vi "flash_lamp (SubVI).vi"(0 "Pulse amp (V)":dbl, 1 "# Pulses in":i32, 2 "Output channel (for flashing)":tag) -> ()   [LabVIEW 2016]
uses:
  <vilib>/DAQmx/write.llb/DAQmx Write (Analog DBL 1Chan 1Samp).vi
  <vilib>/DAQmx/write.llb/DAQmx Write (Analog 1D DBL 1Chan NSamp).vi
  <vilib>/DAQmx/create/channels.llb/DAQmx Create Channel (AO-Voltage-Basic).vi
  <vilib>/DAQmx/configure/timing.llb/DAQmx Timing (Sample Clock).vi
  <vilib>/DAQmx/miscellaneous.llb/DAQmx Fill In Error Info.vi
panel:
  out "Waveform Graph":dbl[](graph)
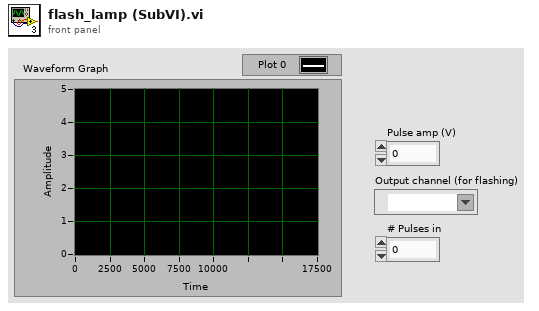
[diagram p1: front panel]
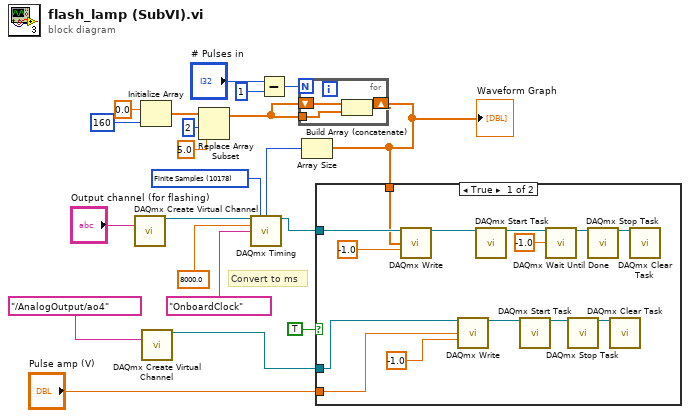
[diagram p0: block diagram]
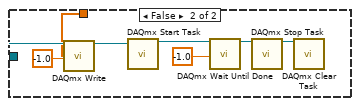
[diagram p2: hidden frame]
diagram:
  w12 = 10178 items=["Finite Samples"=10178, "Continuous Samples"=10123, "Hardware Timed Single Point"=12522] ("sample mode")
  # "Convert to ms"
  n1 = call-poly <vilib>:"DAQmx Create Virtual Channel.vi"("physical channels"="Output channel (for flashing)") -> ("task out"=w20:refnum<k21>)  [unwired: 13 in, 1 out]
  n2 = Initialize Array(0.0 ("element"), 160 ("y")) -> (w6:dbl[])
  n3 = call-poly <vilib>:"DAQmx Create Virtual Channel.vi"("physical channels"=tag "/AnalogOutput/ao4" ("Output channel (for flashing)")) -> ("task out"=w3:refnum<k21>)  [unwired: 13 in, 1 out]
  n4 = Replace Array Subset(array=w6, new element=5.0 ("new element/subarray"), index=2) -> (w14:dbl[])
  n5 = Subtract(x="# Pulses in", y=1) -> (x-y=w5:i32)
  n6 = for {
    N: w5 -> [_]
    shift-right: [w22] -> w7
    shift-left: w14 -> [w24]
    tunnel: w14 -> [w23]
    n7 = Build Array (concatenate)(w24, w23) -> (w22:dbl[])
  }
  "Waveform Graph" <- w7
  n8 = Array Size(array=w7) -> (size(s)=w11:i32)
  n9 = call-poly <vilib>:"DAQmx Timing.vi"("task/channels in"=w20, "sample mode"=w12, "samples per channel"=w11, "rate"=8000.0 ("Sample Rate"), "source"=tag "OnboardClock") -> ("task out"=w18:refnum<k21>)  [unwired: 9 in, 1 out]
  n10 = case shown="True" TRUE {
    tunnel: w18 -> [w32 w44]
    tunnel: w7 -> [w31 w43]
    tunnel: "Pulse amp (V)" -> [w28 _]
    tunnel: w3 -> [w27 _]
    frame True {
      n11 = call-poly <vilib>:"DAQmx Write.vi"("task/channels in"=w32, "data"=w31, "timeout"=-1.0) -> ("task out"=w37:refnum<k21>)  [unwired: 10 in, 2 out]
      n12 = call-poly <vilib>:"DAQmx Write.vi"("task/channels in"=w27, "data"=w28, "timeout"=-1.0) -> ("task out"=w30:refnum<k21>)  [unwired: 10 in, 2 out]
      n13 = call <vilib>:"DAQmx Start Task.vi"("task/channels in"=w37) -> ("task out"=w36:refnum<k21>)  [unwired: 13 in, 1 out]
      n14 = call <vilib>:"DAQmx Start Task.vi"("task/channels in"=w30) -> ("task out"=w25:refnum<k21>)  [unwired: 13 in, 1 out]
      n15 = call <vilib>:"DAQmx Wait Until Done.vi"("task/channels in"=w36, "timeout (sec)"=-1.0) -> ("task out"=w35:refnum<k21>)  [unwired: 12 in, 1 out]
      n16 = call <vilib>:"DAQmx Stop Task.vi"("task/channels in"=w25) -> ("task out"=w26:refnum<k21>)  [unwired: 13 in, 1 out]
      n17 = call <vilib>:"DAQmx Stop Task.vi"("task/channels in"=w35) -> ("task out"=w38:refnum<k21>)  [unwired: 13 in, 1 out]
      n18 = call <vilib>:"DAQmx Clear Task.vi"("task in"=w26) -> ()  [unwired: 14 in, 1 out]
      n19 = call <vilib>:"DAQmx Clear Task.vi"("task in"=w38) -> ()  [unwired: 14 in, 1 out]
    }
    frame False {
      n20 = call-poly <vilib>:"DAQmx Write.vi"("task/channels in"=w44, "data"=w43, "timeout"=-1.0) -> ("task out"=w46:refnum<k21>)  [unwired: 10 in, 2 out]
      n21 = call <vilib>:"DAQmx Start Task.vi"("task/channels in"=w46) -> ("task out"=w39:refnum<k21>)  [unwired: 13 in, 1 out]
      n22 = call <vilib>:"DAQmx Wait Until Done.vi"("task/channels in"=w39, "timeout (sec)"=-1.0) -> ("task out"=w41:refnum<k21>)  [unwired: 12 in, 1 out]
      n23 = call <vilib>:"DAQmx Stop Task.vi"("task/channels in"=w41) -> ("task out"=w40:refnum<k21>)  [unwired: 13 in, 1 out]
      n24 = call <vilib>:"DAQmx Clear Task.vi"("task in"=w40) -> ()  [unwired: 14 in, 1 out]
    }
  }
